vi "mainUIWholeBrainImager.vi"() -> ()   [LabVIEW 2017]
uses:
  globalUtilities.vi
  globalDevices.vi
panel:
  out "duration of recording":string
  out "volumesSaved":i32
  out "frameSaved":u32
  out "frameBrightness":dbl[](graph)
  out "frame":u16[][](graph)
  in  "autofocus":bool
  out "framesNotRead":i32
  out "framesNotSaved":i32
  in  "saveFrames":bool
  in  "saveVolume":bool
  out "YZ":u8[][](graph)
  out "XY":u8[][](graph)
  out "volumes acquired":i32
  in  "STOP":bool
  out "folder name":string
  in  "frames per second":dbl=200.0
  in  "GUI update divider":i32=16
  in  "volumes per second":dbl=3.0
  in  "volume height (um)":dbl=80.0
  # "WHOLE BRAIN IMAGER"
  # "Acquisition parameters"
  # "X on xbox controller"
  # "B on xbox controller\nStarts recording\nframes continuously"
  # "(1/2 the actual frequency)"
  # "flash: Y on xbox controller"
  # "Diagnostics"
  # "Saves one single\nvolume to a separate\nfile."
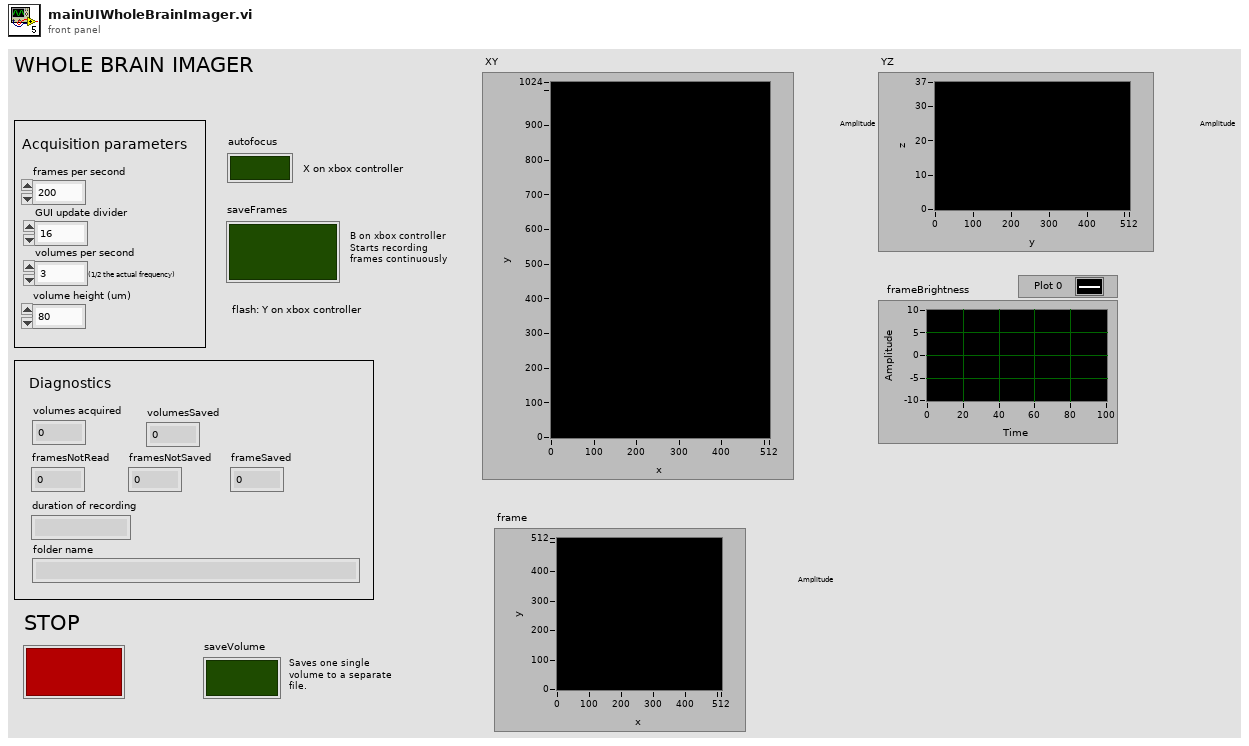
[diagram p1: front panel]
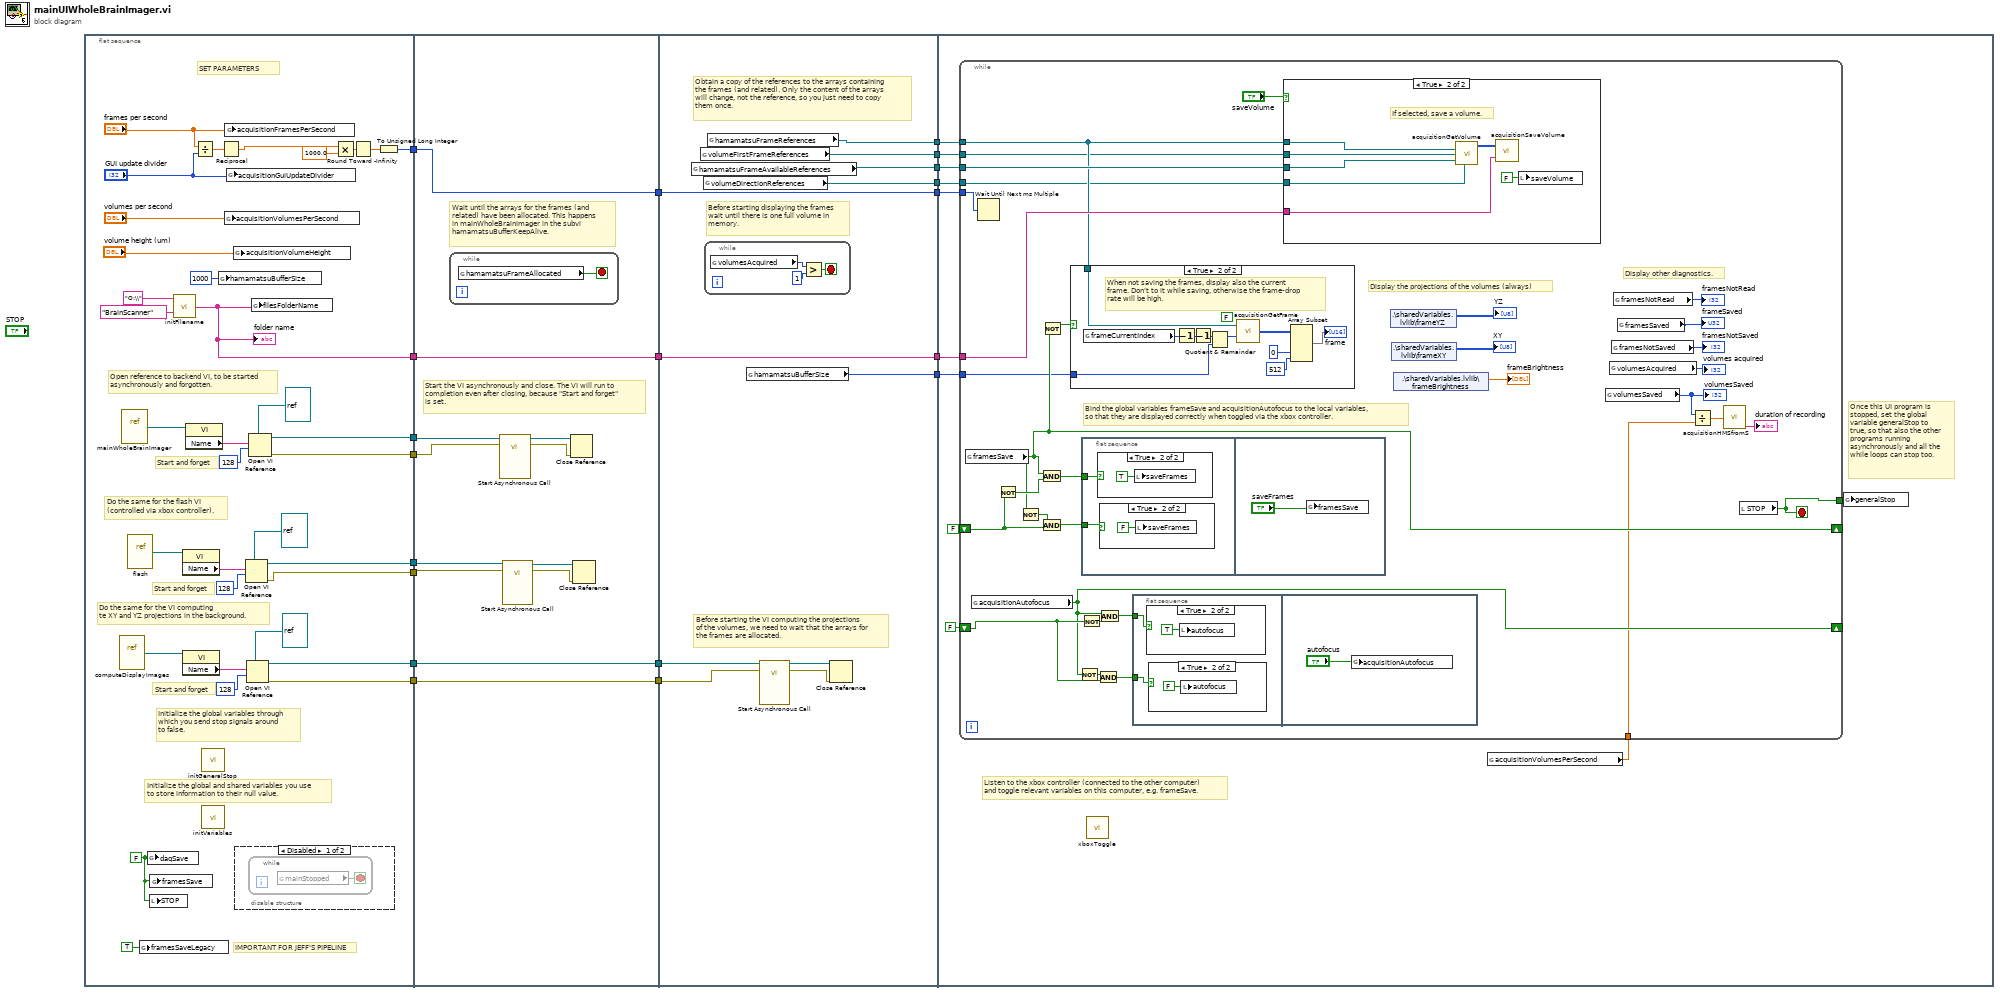
[diagram p0: block diagram]
diagram:
  n1 = flat-sequence {
    tunnel: [w48] -> w19
    tunnel: [w43] -> w18
    tunnel: [w42] -> w17
    tunnel: [w34] -> w14
    tunnel: [w33] -> w13
    tunnel: [w28] -> w10
    tunnel: [w21] -> w6
    tunnel: [w20] -> w4
    tunnel: w19 -> [w66]
    tunnel: w18 -> [w63]
    tunnel: w17 -> [w62]
    tunnel: [w66] -> w16
    tunnel: w14 -> [w60]
    tunnel: w13 -> [w59]
    tunnel: w10 -> [w57]
    tunnel: [w57] -> w8
    tunnel: [w56] -> w7
    tunnel: w6 -> [w56]
    tunnel: [w55] -> w5
    tunnel: w4 -> [w55]
    tunnel: w16 -> [w78]
    tunnel: [w78] -> w15
    tunnel: [w77] -> w12
    tunnel: [w76] -> w11
    tunnel: [w75] -> w9
    tunnel: w8 -> [w75]
    tunnel: w7 -> [w72]
    tunnel: w5 -> [w71]
    tunnel: [w70] -> w3
    tunnel: [w69] -> w2
    tunnel: [w68] -> w1
    tunnel: w15 -> [w92]
    tunnel: w12 -> [w87]
    tunnel: w11 -> [w88]
    tunnel: w9 -> [w90]
    tunnel: w3 -> [w86]
    tunnel: w2 -> [w85]
    tunnel: w1 -> [w84]
    frame #0 {
      w40 = FALSE ("daqSave")
      # "Initialize the global and shared variables you use\nto store information to their null value."
      # "Initialize the global variables through\nwhich you send stop signals around\nto false."
      # "Do the same for the VI computing\nte XY and YZ projections in the background."
      # "Start and forget"
      # "Start and forget"
      # "Do the same for the flash VI \n(controlled via xbox controller)."
      # "IMPORTANT FOR JEFF'S PIPELINE"
      # "Start and forget"
      # "Open reference to backend VI, to be started\nasynchronously and forgotten."
      # "SET PARAMETERS"
      n2 = vi-ref "computeDisplayImages.vi"() -> (w22:refnum<vi>)
      n3 = vi-ref "mainWholeBrainImager.vi"() -> (w41:refnum<vi>)
      n4 = vi-ref "flash.vi"() -> (w35:refnum<vi>)
      n5 = global write "globalUtilities.vi" "framesSaveLegacy"(TRUE ("framesSaveLegacy")) -> ()
      n6 = global write "globalUtilities.vi" "daqSave"(w40) -> ()
      n7 = local write "STOP"(w40) -> ()
      n8 = global write "globalUtilities.vi" "framesSave"(w40) -> ()
      n9 = call "initFilename.vi"("Experiment type"="BrainScanner", "Base disk and folder"="O:\\") -> ("folder name"=w48:string)
      "folder name" <- w48
      n10 = property class="VI"(reference=w35) -> ("Name"=w36:string)  [unwired: 1 in, 2 out]
      n11 = property class="VI"(reference=w22) -> ("Name"=w25:string)  [unwired: 1 in, 2 out]
      n12 = property class="VI"(reference=w41) -> ("Name"=w46:string)  [unwired: 1 in, 2 out]
      n13 = Divide(x="frames per second", y="GUI update divider") -> (x/y=w53:dbl)
      n14 = call "initGeneralStop.vi"() -> ()  [unwired: 1 in]
      n15 = call "initVariables.vi"() -> ()  [unwired: 12 in]
      n16 = global write "globalDevices.vi" "hamamatsuBufferSize"(1000 ("hamamatsuBufferSize")) -> ()
      n17 = Reciprocal(x=w53) -> (1/x=w31:dbl)
      n18 = global write "globalUtilities.vi" "acquisitionVolumesPerSecond"("volumes per second") -> ()
      n19 = global write "globalUtilities.vi" "acquisitionFramesPerSecond"("frames per second") -> ()
      n20 = global write "globalUtilities.vi" "acquisitionGuiUpdateDivider"("GUI update divider") -> ()
      n21 = global write "globalUtilities.vi" "acquisitionVolumeHeight"("volume height (um)") -> ()
      n22 = disable-structure shown="Disabled" {
        frame Disabled {
          n23 = while {
            stop <- w54 stop-if-true
            n24 = global read "globalUtilities.vi" "mainStopped"() -> (w54:bool)
          }
        }
        frame Enabled {
        }
      }
      n25 = Open VI Reference(type specifier VI Refnum (for type only)=refnum<vi> refnum, vi path=w36, options=128) -> (vi reference=w34:refnum<vi>, error out=w33:errorcluster)  [unwired: 3 in]
      n26 = Open VI Reference(type specifier VI Refnum (for type only)=refnum<vi> refnum, vi path=w25, options=128) -> (vi reference=w21:refnum<vi>, error out=w20:errorcluster)  [unwired: 3 in]
      n27 = Open VI Reference(type specifier VI Refnum (for type only)=refnum<vi> refnum, vi path=w46, options=128) -> (vi reference=w43:refnum<vi>, error out=w42:errorcluster)  [unwired: 3 in]
      n28 = global write "globalUtilities.vi" "filesFolderName"(w48) -> ()
      n29 = Multiply(x=w31, y=1000.0) -> (x*y=w32:dbl)
      n30 = Round Toward -Infinity(1:w32) -> (0:w29:dbl)
      n31 = To Unsigned Long Integer(number=w29) -> (unsigned 32bit integer=w28:u32)
    }
    frame #1 {
      # "Wait until the arrays for the frames (and\nrelated) have been allocated. This happens\nin mainWholeBrainImager in the subvi \nhamamatsuBufferKeepAlive."
      # "Start the VI asynchronously and close. The VI will run to\ncompletion even after closing, because \"Start and forget\"\nis set."
      n32 = while {
        stop <- w67 stop-if-true
        n33 = global read "globalDevices.vi" "hamamatsuFrameAllocated"() -> (w67:bool)
      }
      n34 = call-by-ref "Start Asynchronous Call"(reference=w63, error in=w62) -> (reference out=w65:refnum<vi>, error out=w64:errorcluster)  [unwired: 12 in]
      n35 = call-by-ref "Start Asynchronous Call"(reference=w60, error in=w59) -> (reference out=w58:refnum<vi>, error out=w61:errorcluster)  [unwired: 12 in]
      n36 = Close Reference(reference=w65, error in (no error)=w64) -> ()  [unwired: 1 out]
      n37 = Close Reference(reference=w58, error in (no error)=w61) -> ()  [unwired: 1 out]
    }
    frame #2 {
      # "Obtain a copy of the references to the arrays containing \nthe frames (and related). Only the content of the arrays\nwill change, not the reference, so you just need to copy\nthem once."
      # "Before starting displaying the frames\nwait until there is one full volume in\nmemory."
      # "Before starting the VI computing the projections\nof the volumes, we need to wait that the arrays for\nthe frames are allocated."
      n38 = global read "globalDevices.vi" "hamamatsuFrameAvailableReferences"() -> (w76:refnum<data-value>[])
      n39 = global read "globalUtilities.vi" "volumeFirstFrameReferences"() -> (w69:refnum<data-value>[])
      n40 = global read "globalUtilities.vi" "volumeDirectionReferences"() -> (w68:refnum<data-value>[])
      n41 = while {
        stop <- w80 stop-if-true
        n42 = global read "globalUtilities.vi" "volumesAcquired"() -> (w79:i32)
        n43 = Greater?(x=w79, y=1) -> (0:w80:bool)
      }
      n44 = global read "globalDevices.vi" "hamamatsuFrameReferences"() -> (w77:refnum<data-value>[])
      n45 = global read "globalDevices.vi" "hamamatsuBufferSize"() -> (w70:i32)
      n46 = call-by-ref "Start Asynchronous Call"(reference=w72, error in=w71) -> (reference out=w74:refnum<vi>, error out=w73:errorcluster)  [unwired: 12 in]
      n47 = Close Reference(reference=w74, error in (no error)=w73) -> ()  [unwired: 1 out]
    }
    frame #3 {
      # "Listen to the xbox controller (connected to the other computer)\nand toggle relevant variables on this computer, e.g. frameSave."
      # "Once this UI program is\nstopped, set the global\nvariable generalStop to\ntrue, so that also the other\nprograms running\nasynchronously and all the\nwhile loops can stop too."
      n48 = call "xboxToggle.vi"() -> ()  [unwired: 12 in]
      n49 = global read "globalUtilities.vi" "acquisitionVolumesPerSecond"() -> (w82:dbl)
      n50 = while {
        tunnel: w92 -> [w125]
        tunnel: [w124] -> w91
        tunnel: w90 -> [w123]
        shift-right: [w109] -> _
        shift-left: FALSE -> [w117]
        tunnel: w88 -> [w114]
        tunnel: w87 -> [w110]
        tunnel: w86 -> [w107]
        tunnel: w85 -> [w106]
        tunnel: w84 -> [w105]
        shift-right: [w100] -> _
        shift-left: FALSE -> [w102]
        tunnel: w82 -> [w95]
        stop <- w124 stop-if-true
        # "Bind the global variables frameSave and acquisitionAutofocus to the local variables, \nso that they are displayed correctly when toggled via the xbox controller."
        # "Display other diagnostics."
        # "Display the projections of the volumes (always)"
        n51 = global read "globalUtilities.vi" "framesSave"() -> (w109:bool)
        n52 = global read "globalUtilities.vi" "acquisitionAutofocus"() -> (w100:bool)
        n53 = Wait Until Next ms Multiple(millisecond multiple=w123) -> ()  [unwired: 1 out]
        n54 = Not(x=w117) -> (.not. x?=w120:bool)
        n55 = Not(x=w109) -> (.not. x?=w118:bool)
        n56 = And(x=w109, y=w120) -> (x .and. y?=w119:bool)
        n57 = And(x=w118, y=w117) -> (x .and. y?=w116:bool)
        n58 = Not(x=w109) -> (.not. x?=w108:bool)
        n59 = case shown="True" w108 {
          tunnel: w110 -> [_ w140]
          tunnel: w107 -> [_ w134]
          frame False {
          }
          frame True {
            (unwired) FALSE ("resize")
            # "When not saving the frames, display also the current\nframe. Don't to it while saving, otherwise the frame-drop\nrate will be high."
            n60 = global read "globalUtilities.vi" "frameCurrentIndex"() -> (w132:i32)
            n61 = Decrement(x=w132) -> (x-1=w135:i32)
            n62 = Decrement(x=w135) -> (x-1=w131:i32)
            n63 = Quotient & Remainder(x=w131, y=w134) -> (x-y*floor(x/y)=w133:i32)  [unwired: 1 out]
            n64 = call "acquisitionGetFrame.vi"("index"=w133, "hamamatsuFrameReferences"=w140) -> ("frameOut"=w139:u16[][])
            n65 = Array Subset(array=w139, index (col)=0 ("index"), length (col)=512 ("length")) -> (→"frame":u16[][])  [unwired: 2 in]
          }
        }
        n66 = Not(x=w100) -> (.not. x?=w99:bool)
        n67 = Not(x=w102) -> (.not. x?=w104:bool)
        n68 = flat-sequence {
          tunnel: w119 -> [w149]
          tunnel: w116 -> [w148]
          frame #0 {
            n69 = case shown="True" w149 {
              frame False {
              }
              frame True {
                n70 = local write "saveFrames"(TRUE ("saveFrames")) -> ()
              }
            }
            n71 = case shown="True" w148 {
              frame False {
              }
              frame True {
                n72 = local write "saveFrames"(FALSE ("saveFrames")) -> ()
              }
            }
          }
          frame #1 {
            n73 = global write "globalUtilities.vi" "framesSave"("saveFrames") -> ()
          }
        }
        n74 = And(x=w99, y=w102) -> (x .and. y?=w101:bool)
        n75 = And(x=w100, y=w104) -> (x .and. y?=w103:bool)
        n76 = flat-sequence {
          tunnel: w103 -> [w127]
          tunnel: w101 -> [w126]
          frame #0 {
            n77 = case shown="True" w127 {
              frame False {
              }
              frame True {
                n78 = local write "autofocus"(TRUE ("autofocus")) -> ()
              }
            }
            n79 = case shown="True" w126 {
              frame False {
              }
              frame True {
                n80 = local write "autofocus"(FALSE ("autofocus")) -> ()
              }
            }
          }
          frame #1 {
            n81 = global write "globalUtilities.vi" "acquisitionAutofocus"("autofocus") -> ()
          }
        }
        n82 = case shown="True" "saveVolume" {
          tunnel: w125 -> [_ w147]
          tunnel: w114 -> [_ w145]
          tunnel: w110 -> [_ w144]
          tunnel: w106 -> [_ w142]
          tunnel: w105 -> [_ w141]
          frame False {
          }
          frame True {
            # "If selected, save a volume."
            n83 = call "acquisitionGetVolume.vi"("volumeDirectionReferences"=w141, "hamamatsuFrameAvailableReferences"=w145, "volumeFirstFrameReferences"=w142, "hamamatsuFrameReferences"=w144) -> ("volume out"=w143:u16[][][])  [unwired: 1 in, 4 out]
            n84 = call "acquisitionSaveVolume.vi"("folder"=w147, "volume"=w143) -> ()  [unwired: 1 in]
            n85 = local write "saveVolume"(FALSE ("saveVolume")) -> ()
          }
        }
        n86 = shared-variable ".\\sharedVariables.lvlib\\frameYZ"() -> (→"YZ":u8[][])  [unwired: 1 in, 1 out]
        n87 = shared-variable ".\\sharedVariables.lvlib\\frameXY"() -> (→"XY":u8[][])  [unwired: 1 in, 1 out]
        n88 = shared-variable ".\\sharedVariables.lvlib\\frameBrightness"() -> (→"frameBrightness":dbl[])  [unwired: 1 in, 1 out]
        n89 = global read "globalUtilities.vi" "volumesSaved"() -> (w96:i32)
        "volumesSaved" <- w96
        n90 = global read "globalUtilities.vi" "volumesAcquired"() -> (→"volumes acquired":i32)
        n91 = global read "globalUtilities.vi" "framesNotSaved"() -> (→"framesNotSaved":i32)
        n92 = global read "globalUtilities.vi" "framesNotRead"() -> (→"framesNotRead":i32)
        n93 = global read "globalUtilities.vi" "framesSaved"() -> (→"frameSaved":u32)
        n94 = Divide(x=w96, y=w95) -> (x/y=w94:dbl)
        n95 = call "acquisitionHMSfromS.vi"("seconds"=w94) -> ("formatted string"=→"duration of recording":string)  [unwired: 3 out]
        n96 = local read "STOP"() -> (w124:bool)
      }
      n97 = global write "globalUtilities.vi" "generalStop"(w91) -> ()
    }
  }
